vi "RefreshAllObjects.vi"(8 "error in (no error)":errorcluster, 10 "Refresh":T1, 11 "Setting Database in":refnum<class "Setting Database.lvclass">) -> (0 "error out":errorcluster, 3 "Setting Database out":refnum<class "Setting Database.lvclass">)   [LabVIEW 2019, in "Setting Database.lvclass"]
uses:
  Setting Database.lvclass
  Typedefs/PrivateEvents--Setting Database.Refresh.ctl
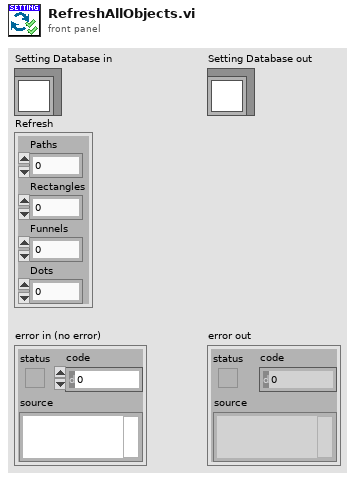
[diagram p1: front panel]
types:
  T1 = typedef "Setting Database.lvclass/PrivateEvents--Setting Database.Refresh.ctl" = cluster{"Paths":i32, "Rectangles":i32, "Funnels":i32, "Dots":i32}
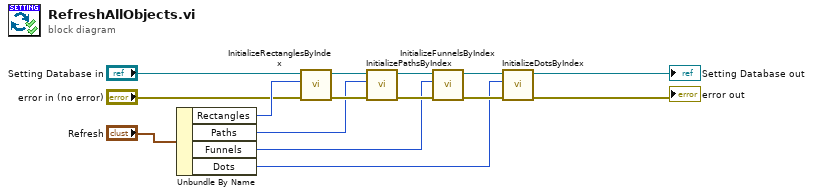
[diagram p0: block diagram]
diagram:
  n1 = Unbundle By Name("Refresh") -> ("Rectangles"=w10:i32, "Paths"=w9:i32, "Funnels"=w8:i32, "Dots"=w5:i32)
  n2 = call "InitializeRectanglesByIndex.vi"("error in (no error)"="error in (no error)", "Index"=w10, "Setting Database in"="Setting Database in") -> ("error out"=w14:errorcluster, "Setting Database out"=w15:refnum<class "Setting Database.lvclass">)  [unwired: 7 in]
  n3 = call "InitializePathsByIndex.vi"("error in (no error)"=w14, "Index"=w9, "Setting Database in"=w15) -> ("error out"=w12:errorcluster, "Setting Database out"=w13:refnum<class "Setting Database.lvclass">)  [unwired: 7 in]
  n4 = call "InitializeFunnelsByIndex.vi"("error in (no error)"=w12, "Index"=w8, "Setting Database in"=w13) -> ("error out"=w6:errorcluster, "Setting Database out"=w7:refnum<class "Setting Database.lvclass">)  [unwired: 7 in]
  n5 = call "InitializeDotsByIndex.vi"("error in (no error)"=w6, "Index"=w5, "Setting Database in"=w7) -> ("error out"=→"error out":errorcluster, "Setting Database out"=→"Setting Database out":refnum<class "Setting Database.lvclass">)  [unwired: 7 in]
